vi "Do.vi"(8 "error in (no error)":errorcluster, 10 "Actor in":refnum<class "Actor.lvclass">, 11 "Bus Monitor Notification Msg":refnum<class "Bus Monitor Notification Msg.lvclass">) -> (0 "error out":errorcluster, 2 "Actor out":refnum<class "Actor.lvclass">)   [LabVIEW 2017, in "Mediator.lvlib" / "Bus Monitor Notification Msg.lvclass"]
doc: "(<B>Filename</B>: Actor Framework.lvlib:Message.lvclass:Do.vi)\n\nDefines what a message does when it is received by an actor. Generally, a message instructs an actor to invoke one of its methods. By default, this method does nothing. A child class must override it to define behavior. Create a child class by using the Actor Framework Message Maker dialog box."
uses:
  Bus Monitor Notification Msg.lvclass
  C:/Git/mva-framework/Source/Framework/Transport/ActorMessageTransport/Notification Msg/Notification Msg.lvclass
  <vilib>/ActorFramework/Actor/Actor.lvclass
  MediatorBusMonitor/MediatorBusMonitor.lvclass
  C:/Program Files (x86)/National Instruments/LabVIEW 2017/vi.lib/ActorFramework/Actor/Actor.lvclass
  Transport/ActorMessageTransport/Notification Msg/Notification Msg.lvclass/Notification Msg.ctl
  Transport/ActorMessageTransport/Notification Msg/Notification Msg.lvclass
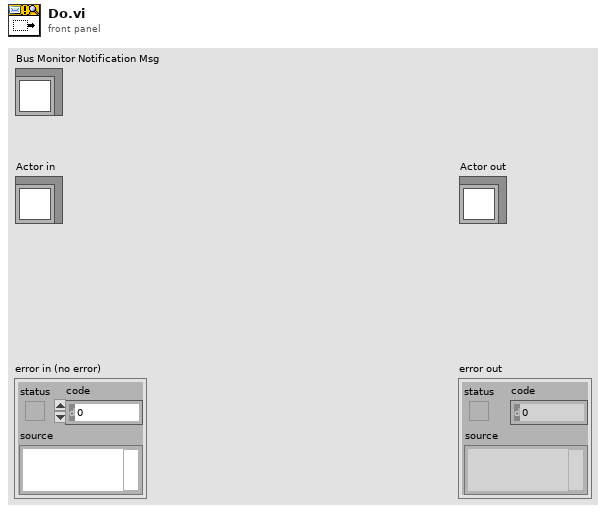
[diagram p1: front panel]
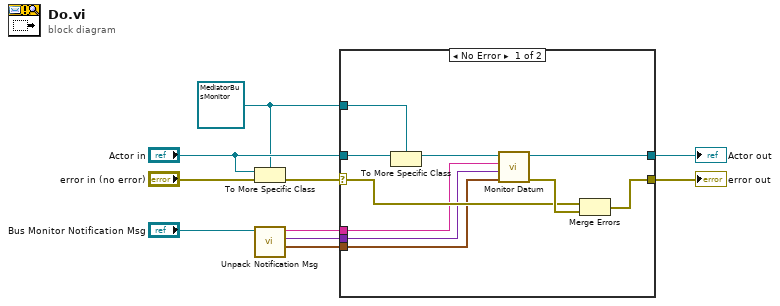
[diagram p0: block diagram]
diagram:
  w1 = refnum<class "MediatorBusMonitor.lvclass"> refnum ("Actor in")
  n1 = To More Specific Class(target class=w1, reference="Actor in", error in="error in (no error)") -> (error out=w10:errorcluster)  [unwired: 1 out]
  n2 = call "Unpack Notification Msg.vi"("Notification Msg"="Bus Monitor Notification Msg") -> ("Publication Time"=w2:timestamp, "Value"=w3:variant, "Datum Name"=w4:string)  [unwired: 8 in]
  n3 = case shown="No Error" w10 {
    selector: w10 -> [w14 w22]
    tunnel: [w15 w22] -> w8
    tunnel: [w17 w21] -> w9
    tunnel: "Actor in" -> [w20 w21]
    tunnel: w1 -> [w19 _]
    tunnel: w4 -> [w13 _]
    tunnel: w3 -> [w12 _]
    tunnel: w2 -> [w11 _]
    frame No Error {
      n4 = To More Specific Class(target class=w19, reference=w20) -> (specific class reference=w18:refnum<class "MediatorBusMonitor.lvclass">)  [unwired: 1 in, 1 out]
      n5 = call "Monitor Datum.vi"("Time Stamp"=w11, "Datum"=w12, "Name"=w13, "MediatorBusMonitor In"=w18) -> ("error out"=w16:errorcluster, "MediatorBusMonitor Out"=w17:refnum<class "MediatorBusMonitor.lvclass">)  [unwired: 6 in]
      n6 = Merge Errors(w14, w16) -> (w15:errorcluster)
    }
    frame Error {
      # "If type check fails, pass the\noriginal object out again."
    }
  }
  "error out" <- w8
  "Actor out" <- w9
